vi "Close All Nested.vi"(8 "error in (no error)":errorcluster, 11 "Module in":refnum<class "Module.lvclass">) -> (0 "error out":errorcluster, 3 "Module out":refnum<class "Module.lvclass">)   [LabVIEW 2020, in "Volatus.lvlib" / "Module.lvclass"]
uses:
  Module.lvclass
  Event Level.ctl
  Module.lvclass/Module.ctl
  MessageQ/MessageQ.lvclass
  Volatus.lvlib
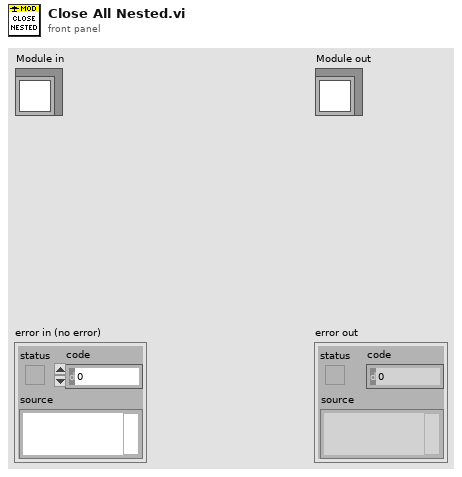
[diagram p1: front panel]
types:
  T1 = typedef "Volatus.lvlib/Module Status.ctl" = cluster{"MessageQ":refnum<class "MessageQ.lvclass">, "State":T2, "Hierarchy":string[], "Forwarded":bool}
  T2 = typedef "Volatus.lvlib/Module.lvclass/State.ctl" = enum16{"Unknown", "Launched", "Starting", "Running", "Stopping", "Stopped", "Error - Starting", "Error - Run", "Error - Stopping"}
  T3 = typedef "Volatus.lvlib/Event Level.ctl" = enum16{"Debug", "Info", "Warning", "Error"}
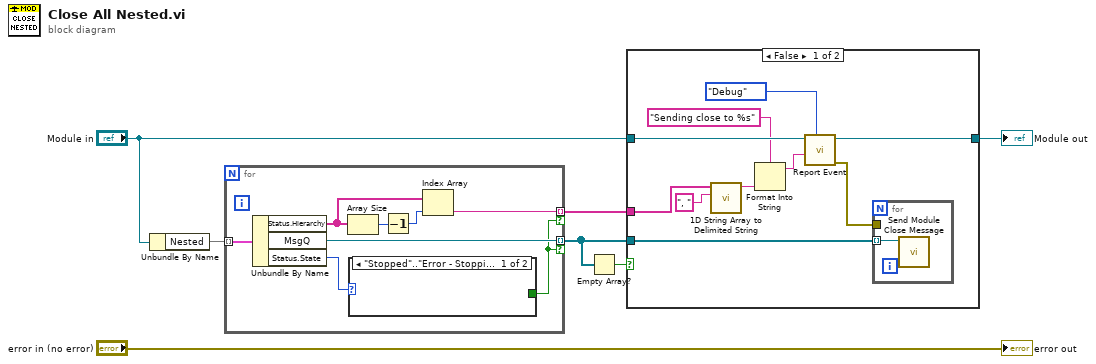
[diagram p0: block diagram]
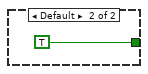
[diagram p2: hidden frame]
diagram:
  n1 = Unbundle By Name("Module in") -> ("Nested"=w5:map{refnum<class "MessageQ.lvclass">, T1})
  n2 = for {
    tunnel: w5 -> [w15] mode=indexing
    tunnel: [w11] -> w2 mode=indexing if=w8
    tunnel: [w9] -> w4 mode=indexing if=w8
    n3 = Unbundle By Name(w15) -> ("Status.Hierarchy"=w12:string[], "MsgQ"=w11:refnum<class "MessageQ.lvclass">, "Status.State"=w14:T2)
    n4 = Array Size(array=w12) -> (size(s)=w13:i32)
    n5 = case shown="\"Stopped\"..\"Error - Stopping\"" w14 {
      tunnel: [_ TRUE] -> w8
      frame "Stopped".."Error - Stopping" {
      }
      frame Default {
      }
    }
    n6 = Decrement(x=w13) -> (x-1=w10:i32)
    n7 = Index Array(array=w12, index=w10) -> (element=w9:string)
  }
  n8 = Empty Array?(array=w2) -> (empty?=w1:bool)
  n9 = case shown="False" w1 {
    tunnel: "Module in" -> [w26 w28]
    tunnel: w4 -> [w25 _]
    tunnel: [w21 w28] -> w3
    tunnel: w2 -> [w18 _]
    frame False {
      n10 = call <vilib>:"1D String Array to Delimited String.vi"("delimiter"=", ", "string array"=w25) -> ("delimited string"=w23:string)  [unwired: 9 in]
      n11 = Format Into String(format string="Sending close to %s", w23) -> (resulting string=w19:string)  [unwired: 2 in, 1 out]
      n12 = call "Report Event.vi"("Level (Info)"=Event_Level."Debug", "Message"=w19, "Module in"=w26) -> ("error out"=w17:errorcluster, "Module out"=w21:refnum<class "Module.lvclass">)  [unwired: 7 in]
      n13 = for {
        tunnel: w18 -> [w27] mode=indexing
        tunnel: w17 -> [_]
        n14 = call "Send Module Close Message.vi"("MessageQ"=w27) -> ()  [unwired: 10 in, 1 out]
      }
    }
    frame True {
    }
  }
  "Module out" <- w3
  "error out" <- "error in (no error)"
